vi "Write Level Value.vi"(8 "error in (no error)":errorcluster, 10 "Level":dbl, 11 "Channel in":refnum<class "Channel.lvclass">) -> (0 "error out":errorcluster, 3 "Channel out":refnum<class "Channel.lvclass">)   [LabVIEW 2020, in "Channel.lvclass"]
uses:
  Channel.lvclass
  Channel.lvclass/Channel.ctl
  Level/Level.lvclass/Level.ctl
  Level/Level.lvclass
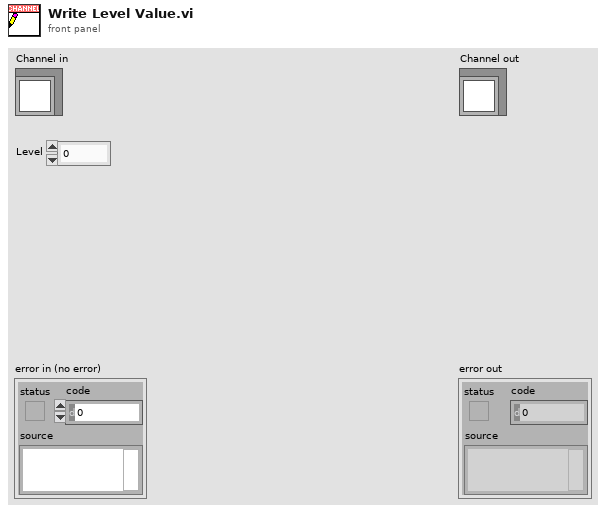
[diagram p1: front panel]
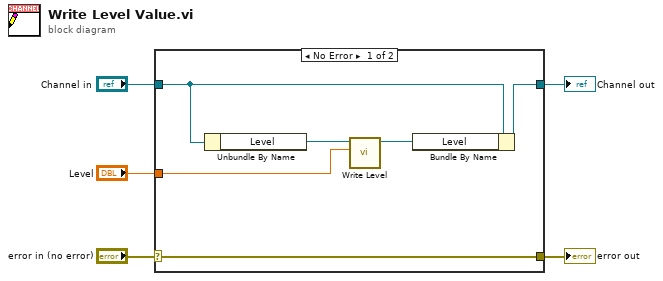
[diagram p0: block diagram]
diagram:
  n1 = case shown="No Error" "error in (no error)" {
    selector: "error in (no error)" -> [w11 w12]
    tunnel: [w11 w12] -> w4
    tunnel: [w10 w13] -> w2
    tunnel: "Channel in" -> [w9 w13]
    tunnel: "Level" -> [w6 _]
    frame No Error {
      n2 = Unbundle By Name(w9) -> ("Level"=w8:refnum<class "Level.lvclass">)
      n3 = call "Write Level.vi"("Level"=w6, "Level in"=w8) -> ("Level out"=w7:refnum<class "Level.lvclass">)  [unwired: 8 in, 1 out]
      n4 = Bundle By Name(cluster=w9, "Level"=w7) -> (w10:refnum<class "Channel.lvclass">)
    }
    frame Error {
    }
  }
  "error out" <- w4
  "Channel out" <- w2
